vi "Check Size (1D Power of 2).vi"(5 "power of 2":i16, 7 "source vi name":string, 8 "error in (no error)":errorcluster, 9 "transfer count":u64 format="%08x bytes", 10 "buffer element count":u64 format="%08x bytes", 11 "Pointer in":refnum<class "Pointer.lvclass">) -> (0 "error out":errorcluster, 1 "transfer count out":u64 format="%08x bytes", 2 "buffer element count out":u64 format="%08x bytes", 3 "Pointer out":refnum<class "Pointer.lvclass">)   [LabVIEW 2016, in "Memory Manager.lvlib" / "Pointer.lvclass"]
uses:
  Pointer.lvclass
  Buffer Underflow.vi
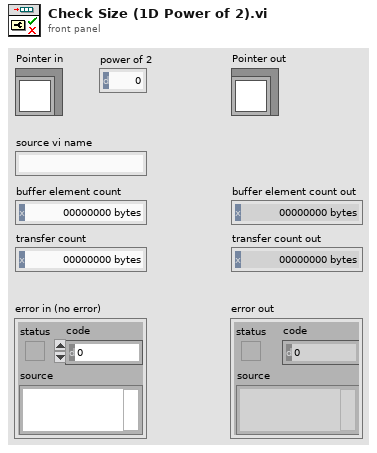
[diagram p1: front panel]
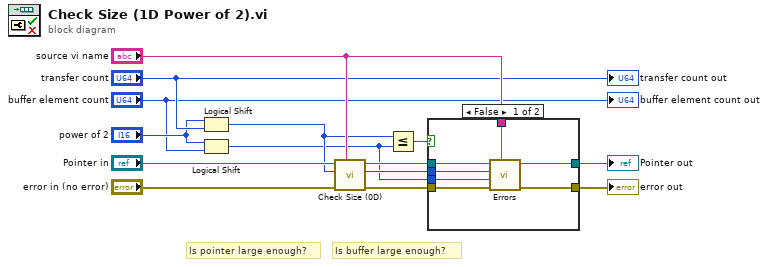
[diagram p0: block diagram]
diagram:
  # "Is buffer large enough?"
  # "Is pointer large enough?"
  n1 = Logical Shift(y="power of 2", x="transfer count") -> (x << y=w4:u64)
  n2 = Logical Shift(y="power of 2", x="buffer element count") -> (x << y=w1:u64)
  n3 = call "Check Size (0D).vi"("source vi name"="source vi name", "error in (no error)"="error in (no error)", "required size"=w4, "Pointer in"="Pointer in") -> ("error out"=w10:errorcluster, "required size out"=w8:u64, "Pointer out"=w11:refnum<class "Pointer.lvclass">)  [unwired: 5 in]
  n4 = Less Or Equal?(x=w4, y=w1) -> (x <= y?=w7:bool)
  n5 = case shown="False" w7 {
    tunnel: w11 -> [w21 w22]
    tunnel: w10 -> [w19 w23]
    tunnel: [w18 w23] -> w14
    tunnel: [w20 w22] -> w13
    tunnel: "source vi name" -> [w17 _]
    tunnel: w1 -> [w16 _]
    tunnel: w8 -> [w15 _]
    frame False {
      n6 = call-poly "Errors.vi"("error source vi name"=w17, "error in (no error)"=w19, "actual buffer size"=w16, "required buffer size"=w15, "Pointer in"=w21) -> ("error out"=w18:errorcluster, "Pointer out"=w20:refnum<class "Pointer.lvclass">)  [unwired: 5 in]
    }
    frame True {
    }
  }
  "error out" <- w14
  "Pointer out" <- w13
  "transfer count out" <- "transfer count"
  "buffer element count out" <- "buffer element count"
